vi "Process GEA Event Dryer.vi"(8 "error in (no error)":errorcluster, 9 "Init Debug File":bool, 10 "Log File Type":T1, 11 "GEA2 Data In":T2 {"Command" format="%02x"; "Destination" format="%02x"; "Source" format="%02x"}) -> (0 "error out":errorcluster, 1 "Debug File Initialized":bool, 2 "End Cycle":bool, 3 "Output String":string)   [LabVIEW 2014]
uses:
  Common/LabVIEW GEA2 Toolkit/LabVIEW_GEA2_Toolkit.lvlibp/type defs/Data In.ctl
  type defs/Log_File_Type.ctl
  Common/LabVIEW GEA2 Toolkit/LabVIEW_GEA2_Toolkit.lvlibp
panel:
  out "Prepend Time Stamp":bool
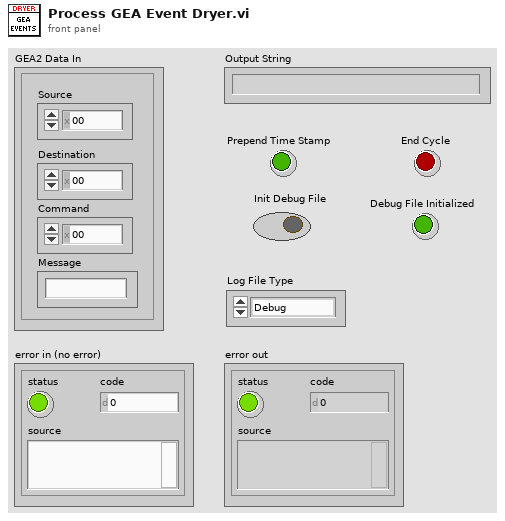
[diagram p1: front panel]
types:
  T1 = typedef "Log_File_Type.ctl" = enum16{"Debug", "Bus Traffic"}
  T2 = typedef "LabVIEW_GEA2_Toolkit.lvlibp/Data In.ctl" = cluster{"Source":u8, "Destination":u8, "Command":u8, "Message":string}
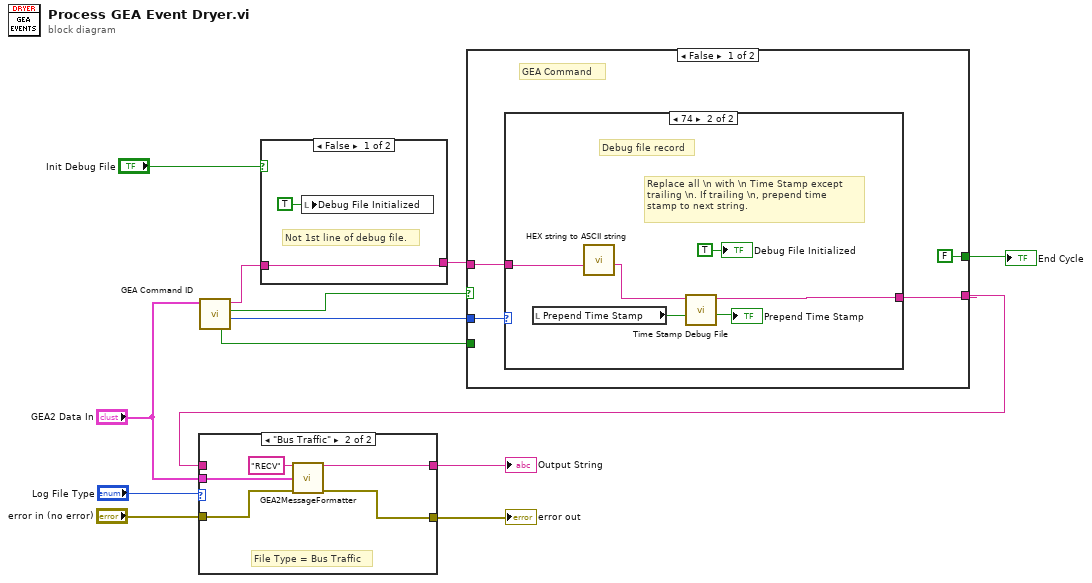
[diagram p0: block diagram]
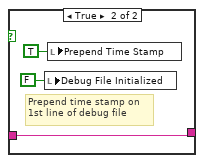
[diagram p2: hidden frame]
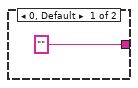
[diagram p3: hidden frame]
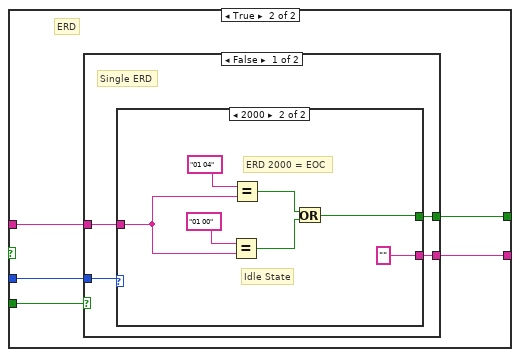
[diagram p4: hidden frame]
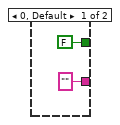
[diagram p5: hidden frame]
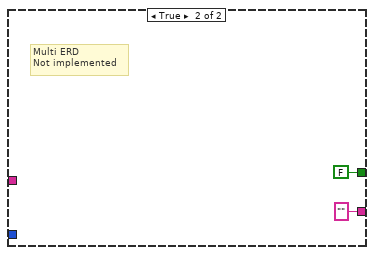
[diagram p6: hidden frame]
diagram:
  n1 = call "GEA Command ID.vi"("GEA2 Data In"="GEA2 Data In") -> ("HEX Command"=w9:u16, "ERD"=w8:bool, "string out"=w2:string, "Multi Command"=w7:bool)  [unwired: 7 in]
  n2 = case shown="False" "Init Debug File" {
    tunnel: w2 -> [w15 w16]
    tunnel: [w15 w16] -> w1
    frame False {
      # "Not 1st line of debug file."
      n3 = local write "Debug File Initialized"(TRUE ("Debug File Initialized")) -> ()
    }
    frame True {
      # "Prepend time stamp on\n1st line of debug file"
      n4 = local write "Debug File Initialized"(FALSE ("Debug File Initialized")) -> ()
      n5 = local write "Prepend Time Stamp"(TRUE ("Prepend Time Stamp")) -> ()
    }
  }
  n6 = case shown="False" w8 {
    tunnel: w9 -> [w21 w34]
    tunnel: w7 -> [_ w33]
    tunnel: w1 -> [w19 w32]
    tunnel: [FALSE w31] -> w6
    tunnel: [w20 w30] -> w5
    frame False {
      # "GEA Command"
      n7 = case shown="74" w21 {
        tunnel: ["" ("Output String") w28] -> w20
        tunnel: w19 -> [_ w29]
        frame 0, Default {
        }
        frame 116 {
          # "Replace all \\n with \\n Time Stamp except\ntrailing \\n. If trailing \\n, prepend time\nstamp to next string."
          # "Debug file record"
          n8 = local read "Prepend Time Stamp"() -> (w25:bool)
          n9 = call "HEX string to ASCII string.vi"("String In"=w29) -> ("String Out"=w27:string)  [unwired: 10 in]
          n10 = call "Time Stamp Debug File.vi"("String In"=w27, "Prepend Stamp"=w25) -> ("result string"=w28:string, "Ends With LF"=→"Prepend Time Stamp":bool)  [unwired: 7 in]
          "Debug File Initialized" <- TRUE ("Debug File Initialized")
        }
      }
    }
    frame True {
      # "ERD"
      n11 = case shown="False" w33 {
        tunnel: w34 -> [w38 _]
        tunnel: w32 -> [w37 _]
        tunnel: [w36 FALSE] -> w31
        tunnel: [w35 "" ("Output String")] -> w30
        frame False {
          # "Single ERD"
          n12 = case shown="2000" w38 {
            tunnel: w37 -> [_ w44]
            tunnel: [FALSE w41] -> w36
            tunnel: ["" ("Output String") "" ("Output String")] -> w35
            frame 0, Default {
            }
            frame 8192 {
              # "Idle State"
              # "ERD 2000 = EOC"
              n13 = Equal?(x="01 00", y=w44) -> (x = y?=w42:bool)
              n14 = Equal?(x="01 04", y=w44) -> (x = y?=w43:bool)
              n15 = Or(x=w43, y=w42) -> (x .or. y?=w41:bool)
            }
          }
        }
        frame True {
          # "Multi ERD\nNot implemented"
        }
      }
    }
  }
  "End Cycle" <- w6
  n16 = case shown="\"Bus Traffic\"" "Log File Type" {
    tunnel: [w50 w56] -> w13
    tunnel: [w51 w55] -> w12
    tunnel: "error in (no error)" -> [w51 w54]
    tunnel: "GEA2 Data In" -> [_ w52]
    tunnel: w5 -> [w50 _]
    frame "Debug", Default {
      # "File Type = Debug"
    }
    frame "Bus Traffic" {
      # "File Type = Bus Traffic"
      n17 = call "GEA2MessageFormatter.vi"("Prefix(Send/Recv)"="RECV", "GEA2 Data In"=w52, "Error In"=w54) -> ("Output String"=w56:string, "Error Out"=w55:errorcluster)  [unwired: 11 in]
    }
  }
  "Output String" <- w13
  "error out" <- w12
